vi "Grava_EQ_registers_u.vi"(3 "EQ Data+Report_u (hex)":u32[](array[numeric]) format="%x", 4 "ChipID (file name)":string, 5 "EQ_u file paths":path[](array[path])) -> ()   [LabVIEW 2015, in "VIPM2.lvlib"]
doc: "Partint del array hex EQ DATA+REPORT d'<b>un sol chip</b>, grava per separat GlobalReg i PixelReg en subcarpetes dedicades."
uses:
  VIPM2.lvlib
panel:
  # "Grava   EQ_GlobalReg_u   i   EQ_PixelReg_u"
  # "EQ_GlobalReg\n\nEQ_PixelReg"
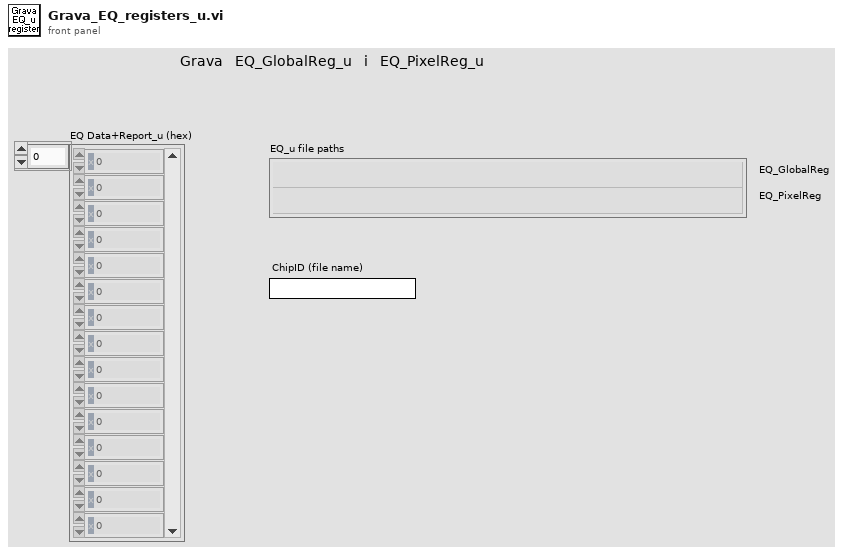
[diagram p1: front panel]
types:
  T1 = enum16{"open", "replace", "create", "open or create", "replace or create", "replace or create with confirmation"}
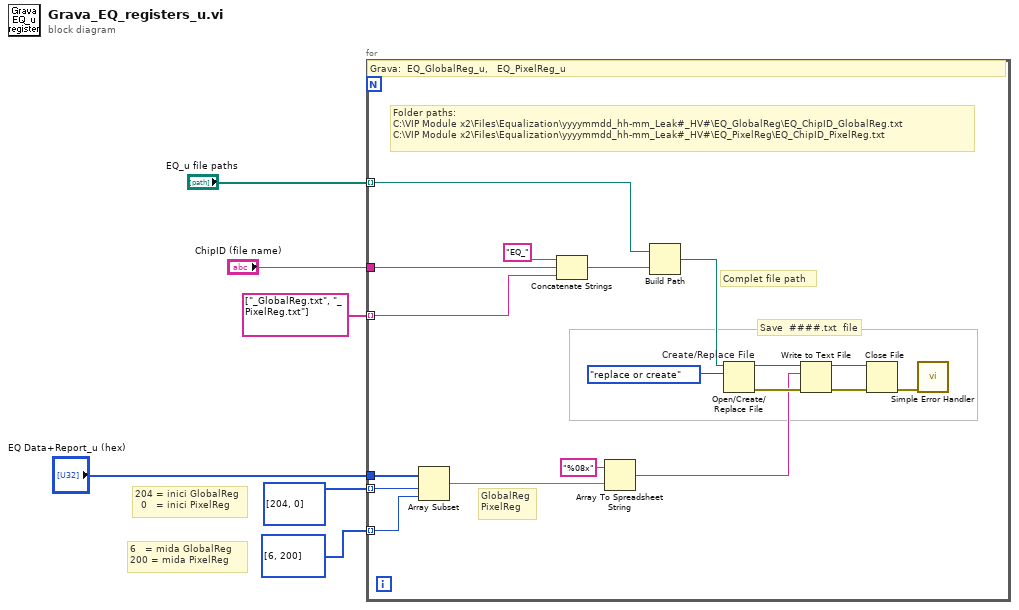
[diagram p0: block diagram]
diagram:
  # "6   = mida GlobalReg\n200 = mida PixelReg"
  # "204 = inici GlobalReg\n  0   = inici PixelReg"
  n1 = for {
    tunnel: "EQ Data+Report_u (hex)" -> [w24]
    tunnel: i32[] [204, 0] -> [w23] mode=indexing
    tunnel: i32[] [6, 200] -> [w22] mode=indexing
    tunnel: "EQ_u file paths" -> [w8] mode=indexing
    tunnel: "ChipID (file name)" -> [w11]
    tunnel: string[] ["_GlobalReg.txt", "_PixelReg.txt"] ("string") -> [w10] mode=indexing
    # "Complet file path"
    # "Save  ####.txt  file"
    # "GlobalReg\nPixelReg"
    # "Folder paths:\nC:\\VIP Module x2\\Files\\Equalization\\yyyymmdd_hh-mm_Leak#_HV#\\EQ_GlobalReg\\EQ_ChipID_GlobalReg.txt\nC:\\VIP Module x2\\Files\\Equalization\\yyyymmdd_hh-mm_Leak#_HV#\\EQ_PixelReg\\EQ_ChipID_PixelReg.txt"
    # "Grava:  EQ_GlobalReg_u,   EQ_PixelReg_u"
    n2 = Array Subset "Array Subset"(array=w24, index=w23, length=w22) -> (w21:u32[])
    n3 = Concatenate Strings "Concatenate Strings"("EQ_" ("string"), w11, w10) -> (w9:string)
    n4 = Array To Spreadsheet String(array=w21, 3:"%08x" ("format string")) -> (spreadsheet string=w13:string)  [unwired: 1 in]
    n5 = Build Path(base path=w8, name or relative path=w9) -> (appended path=w7:path)
    n6 = Open/Create/Replace File "Create/Replace File"(file path (use dialog)=w7, operation (0:open)=T1."replace or create") -> (refnum out=w18:refnum<file>, error out=w17:errorcluster)  [unwired: 4 in, 1 out]
    n7 = Write to Text File(file (use dialog)=w18, text=w13, error in=w17) -> (refnum out=w15:refnum<file>, error out=w16:errorcluster)  [unwired: 1 in, 1 out]
    n8 = Close File(refnum=w15, error in=w16) -> (error out=w14:errorcluster)  [unwired: 1 out]
    n9 = call <vilib>:"Simple Error Handler.vi"("error in (no error)"=w14) -> ()  [unwired: 4 in, 5 out]
  }
